vi "Calibration_Transform.vi"(3 "Conversion Matrix":dbl[][](array[numeric])=[[0.01666666666666666, 0.0, 0.0], [0.0, 0.016666666666666666, 0.0]], 4 "Master CalibrationCoordinates: x,x',y,y'...":dbl[][](array[numeric])=[[0.0, -0.003225, 0.0, 0.001935], [1000.0, 0.003225, 0.0, 0.001935], [0.0, -0.003225, 600.0, -0.001935]]) -> (1 "New CalibrationCoordinates: x,x\",y,y\"...":dbl[][](array[numeric])=[[0.0, 0.0, 0.0, 0.0], [1.0, 1.0, 0.0, 0.0], [0.0, 0.0, 1.0, 1.0]])   [LabVIEW 2011]
panel:
  # "example data is 60x Objective: 1/60x"
  # "x, x-ypart, constant x\ny-xpart, y, constant y"
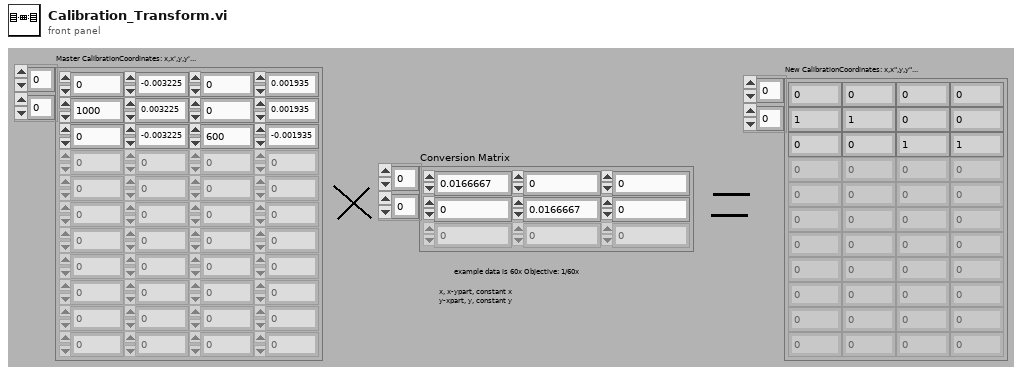
[diagram p1: front panel]
types:
  T1 = cluster{"Master CalibrationCoordinates: x,x',y,y'...[0]":dbl, "Master CalibrationCoordinates: x,x',y,y'...[1]":dbl, "Master CalibrationCoordinates: x,x',y,y'...[2]":dbl, "Master CalibrationCoordinates: x,x',y,y'...[3]":dbl}
  T2 = cluster{"Master CalibrationCoordinates: x,x',y,y'...[1]":dbl, "Master CalibrationCoordinates: x,x',y,y'...[3]":dbl}
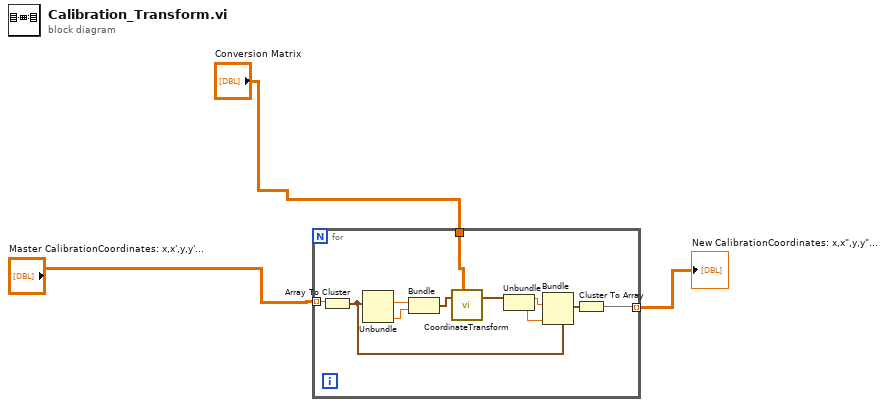
[diagram p0: block diagram]
diagram:
  n1 = for {
    tunnel: "Master CalibrationCoordinates: x,x',y,y'..." -> [w14] mode=indexing
    tunnel: [w5] -> w2 mode=indexing
    tunnel: "Conversion Matrix" -> [w4]
    n2 = Array To Cluster(array=w14) -> (cluster=w13:T1)
    n3 = Unbundle(w13) -> ("Master CalibrationCoordinates: x,x',y,y'...[1]"=w10:dbl, "Master CalibrationCoordinates: x,x',y,y'...[3]"=w9:dbl)  [unwired: 2 out]
    n4 = Bundle("Master CalibrationCoordinates: x,x',y,y'...[1]"=w10, "Master CalibrationCoordinates: x,x',y,y'...[3]"=w9) -> (w11:T2)  [unwired: 1 out]
    n5 = call "CoordinateTransform.vi"("input coordiantes"=w11, "Conversion Matrix"=w4) -> ("output coordiantes"=w12:cluster{"x":dbl, "y":dbl})  [unwired: 2 in, 1 out]
    n6 = Unbundle(w12) -> ("x"=w8:dbl, "y"=w7:dbl)
    n7 = Bundle(cluster=w13, "Master CalibrationCoordinates: x,x',y,y'...[1]"=w8, "Master CalibrationCoordinates: x,x',y,y'...[3]"=w7) -> (w6:T1)  [unwired: 2 out]
    n8 = Cluster To Array(cluster=w6) -> (array=w5:dbl[])
  }
  "New CalibrationCoordinates: x,x\",y,y\"..." <- w2
